vi "Waveform - Common Mathematical Operations.vi"() -> ()   [LabVIEW 2020]
doc: "Shows basic addition, subtraction, multiplication, and division between two waveforms."
panel:
  in  "dt Values":u16(ring) items=["Same", "Different"]
  out "Final Waveform":waveform(dbl)(graph)
  out "Initial Waveforms":waveform(dbl)[](graph)
  in  "Operation":u16(ring) items=["Add", "Subtract", "Multiply", "Divide"]
  # "Overview: Demonstrates the use of the Add, Subtract, Multiply, and Divide functions to perform common mathematical operations on Waveform data types.\nInstructions:\n1. Select an Operation to perform on the waveforms.\n2. Run the VI. The waveforms will be added, subtracted, multiplied, or divided, depending on the Operation you selected.\n3. Change the dt Values to be 'Different'.\n4. Run the VI again. An error is generated because you cannot perform mathematical operations on waveforms with different dt values."
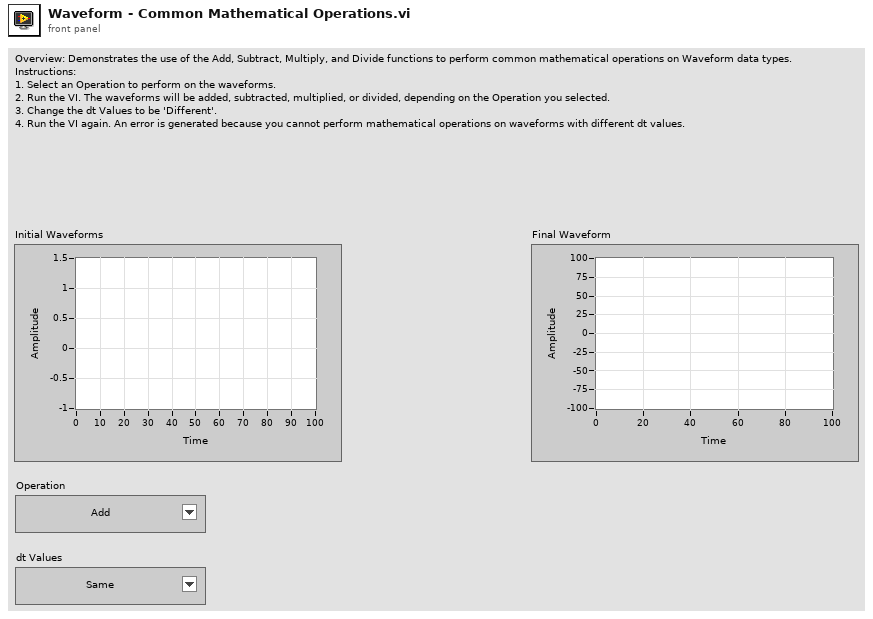
[diagram p1: front panel]
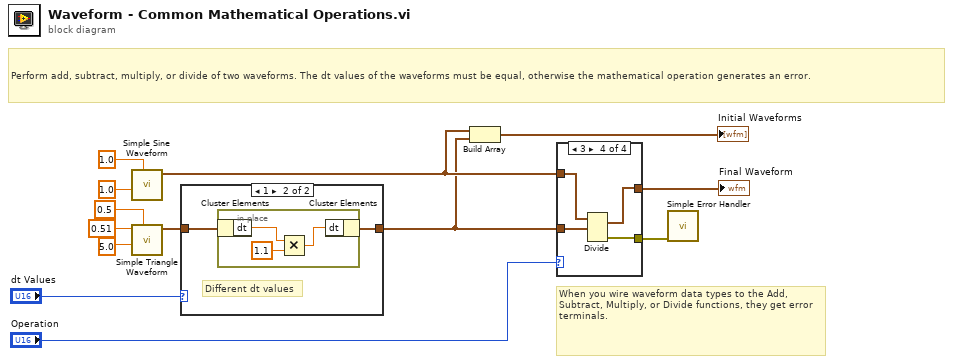
[diagram p0: block diagram]
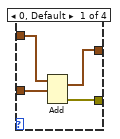
[diagram p3: hidden frame]
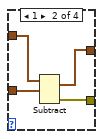
[diagram p4: hidden frame]
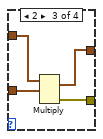
[diagram p5: hidden frame]
diagram:
  # "When you wire waveform data types to the Add, Subtract, Multiply, or Divide functions, they get error terminals."
  # "Perform add, subtract, multiply, or divide of two waveforms. The dt values of the waveforms must be equal, otherwise the mathematical operation generates an error."
  n1 = call "Simple Sine Waveform.vi"("amplitude"=1.0, "n cycles"=1.0) -> ("sine waveform"=w12:waveform(dbl))  [unwired: 9 in]
  n2 = call "Simple Triangle Waveform.vi"("amplitude"=0.5, "n cycles"=5.0, "offset"=0.51) -> ("triangle waveform"=w10:waveform(dbl))  [unwired: 8 in]
  n3 = case shown="1" "dt Values" {
    tunnel: w10 -> [w14 w16]
    tunnel: [w14 w15] -> w9
    frame 0, Default {
      # "Same dt values"
    }
    frame 1 {
      # "Different dt values"
      n4 = in-place {
        n5 = in-place-cluster #1(w16) -> ("dt"=w18:dbl)
        n6 = Multiply(x=w18, y=1.1) -> (x*y=w17:dbl)
        n7 = in-place-cluster #1("dt"=w17) -> (w15:waveform(dbl))
      }
    }
  }
  n8 = Build Array(w12, w9) -> (→"Initial Waveforms":waveform(dbl)[])
  n9 = case shown="3" "Operation" {
    tunnel: w9 -> [w23 w27 w31 w35]
    tunnel: w12 -> [w22 w26 w30 w34]
    tunnel: [w21 w25 w29 w33] -> w1
    tunnel: [w20 w24 w28 w32] -> w11
    frame 0, Default {
      n10 = Add(1:w23, 2:w22) -> (0:w21:waveform(dbl), 3:w20:errorcluster)  [unwired: 1 in]
    }
    frame 1 {
      n11 = Subtract(1:w27, 2:w26) -> (0:w25:waveform(dbl), 3:w24:errorcluster)  [unwired: 1 in]
    }
    frame 2 {
      n12 = Multiply(1:w31, 2:w30) -> (0:w29:waveform(dbl), 3:w28:errorcluster)  [unwired: 1 in]
    }
    frame 3 {
      n13 = Divide(1:w35, 2:w34) -> (0:w33:waveform(dbl), 3:w32:errorcluster)  [unwired: 1 in]
    }
  }
  "Final Waveform" <- w1
  n14 = call <vilib>:"Simple Error Handler.vi"("error in (no error)"=w11) -> ()  [unwired: 4 in, 5 out]
